vi "BasicFPGATest.vi"() -> ()   [LabVIEW 2015]
uses:
  Core/SingleAIConfig.ctl
  Core/ScaleAndLimitAI16Config.ctl
  Core/AI16LimitsConfig.ctl
  Core/AI16ScaleConfig.ctl
  <vilib>/Platform/TimedLoop/XDataNode/timing_clust.ctl
  <vilib>/Platform/TimedLoop/XDataNode/nitl_modes.ctl
  <vilib>/Platform/TimedLoop/XDataNode/wakeup.ctl
  <vilib>/rvi/Emulation/niFpgaGetClockAttributes.vi
  <vilib>/rvi/Emulation/niFpgaSctlEmulationGetInTimedLoop.vi
  <vilib>/rvi/Emulation/niFpgaEmulationReportErrorSimple.vi
  <vilib>/NI/PowerElectronicsControl/Utility/FPGA_Timers/TickTocks/Tick0.vi
  <vilib>/rvi/Emulation/niFpgaCriticalErrorInLSC.vi
  <vilib>/NI/PowerElectronicsControl/Utility/FPGA_Timers/TickTocks/Tock0.vi
  <vilib>/NI/PowerElectronicsControl/Utility/FPGA_Timers/TickTocks/Tick2.vi
  <vilib>/rvi/eio/common/nirviEmuTemplateMethod_errors.vi
  <vilib>/NI/PowerElectronicsControl/Utility/FPGA_Timers/TickTocks/Tock2.vi
  <vilib>/NI/PowerElectronicsControl/Utility/FPGA_Timers/TickTocks/Tick3.vi
  <vilib>/NI/PowerElectronicsControl/Utility/FPGA_Timers/TickTocks/Tock3.vi
  <vilib>/Platform/TimedLoop/XDataNode/XDataNode.xnode
  <vilib>/eio/EIONode/EIONode.xnode
  Core/ScaleAndLimit.lvlib
  <vilib>/Platform/TimedLoop/XDataNode/XDNodeRunTimeDep.lvlib
  <vilib>/NI/PowerElectronicsControl/Utility/FPGA_Timers/Timers.lvlib
panel:
  out "UnscaledAI":i16[](array[numeric])
  in  "DummyAI15":i16
  in  "SingleAIConfig":T1
  in  "loop wait":u32 caption="Count(Ticks)"
  out "scale and fault":u32
  out "I/O":u32
  in  "resetMaxTime":bool
  out "MaxTimes":u32[](array[numeric])
  out "Times":u32[](array[numeric])
  out "AILimitLow":u16 format="%.0x"
  out "AILimitHigh":u16 format="%.0x"
  out "AILimits":bool
  out "ScaledAI":sgl[](array[numeric])
  in  "ClearLimits":bool
  out "loop time":u32
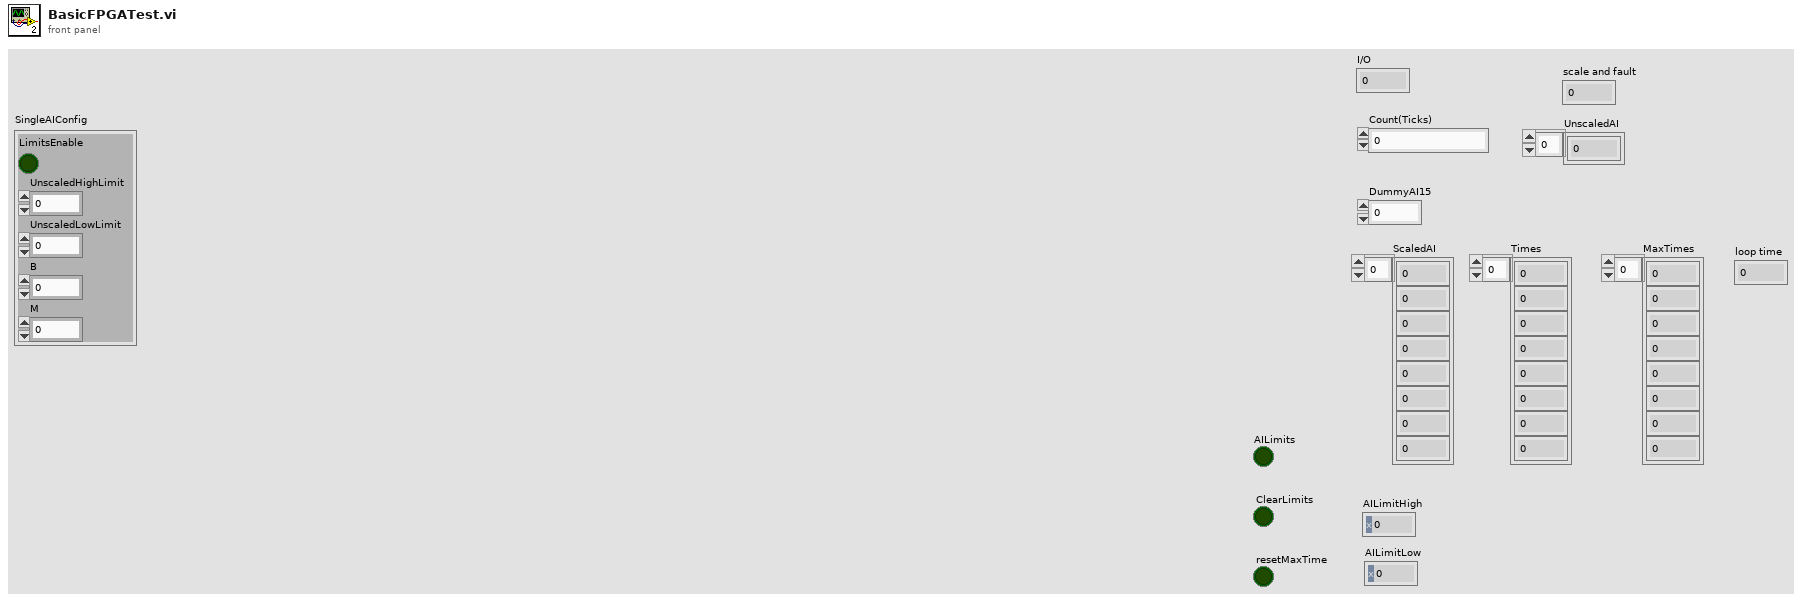
[diagram p1: front panel]
types:
  T1 = typedef "ScaleAndLimit.lvlib/SingleAIConfig.ctl" = cluster{"LimitsEnable":bool, "UnscaledHighLimit":i16, "UnscaledLowLimit":i16, "B":i16, "M":sgl}
  T2 = typedef "ScaleAndLimit.lvlib/ScaleAndLimitAI16Config.ctl" = cluster{"AI16Limits":T3, "AI16ScaleConfig":T4}
  T3 = typedef "ScaleAndLimit.lvlib/AI16LimitsConfig.ctl" = cluster{"LimitsEnabled":u16, "UnscaledHighLimit":i16[], "UnscaledLowLimit":i16[]}
  T4 = typedef "ScaleAndLimit.lvlib/AI16ScaleConfig.ctl" = cluster{"B":i16[], "M":sgl[]}
  T5 = typedef "Timers.lvlib/TimerRegisters.ctl" = cluster{"Tick0":refnum<k21>, "Tock0":refnum<k21>, "Tick1":refnum<k21>, "Tock1":refnum<k21>, "Tick2":refnum<k21>, "Tock2":refnum<k21>, "Tick3":refnum<k21>, "Tock3":refnum<k21>, "Tick4":refnum<k21>, "Tock4":refnum<k21>, "Tick5":refnum<k21>, "Tock5":refnum<k21>, "Tick6":refnum<k21>, "Tock6":refnum<k21>, "Tick7":refnum<k21>, "Tock7":refnum<k21>}
  T6 = typedef "XDNodeRunTimeDep.lvlib/timing_clust.ctl" = cluster{"Expected End [f-1]":u64, "Actual End [f-1]":u64, "Finished Late? [f-1]":bool, "Expected End [i-1]":u64, "Actual End [i-1]":u64, "Finished Late? [i-1]":bool, "Expected Start [i]":u64, "Actual Start [i]":u64, "Expected Start [f]":u64, "Actual Start [f]":u64, "Source Name":string, "Structure Name":string, "Period":i64, "Deadline":i64, "Offset":i64, "Start":i64, "Priority":i32, "Timeout":i32, "Mode":T7, "Wakeup Reason":T8, "Error":errorcluster, "Source Type":string, "Secondary Source Type":string, "Global End Time":u64, "Global Start Time":u64, "Frame Duration":u64, "Iteration Duration":u64, "Assigned CPU":i32, "I/O Scan Engine Mode":u32}
  T7 = typedef "XDNodeRunTimeDep.lvlib/nitl_modes.ctl" = enum32{"No Change", "Process missed periods, maintain original phase", "Discard missed periods, maintain original phase", "Process missed periods, ignore original phase", "Discard missed periods, ignore original phase"}
  T8 = typedef "XDNodeRunTimeDep.lvlib/wakeup.ctl" = enum32{"Normal", "Aborted", "Asynchronous wakeup", "Timing source error", "Timed loop error", "Timeout"}
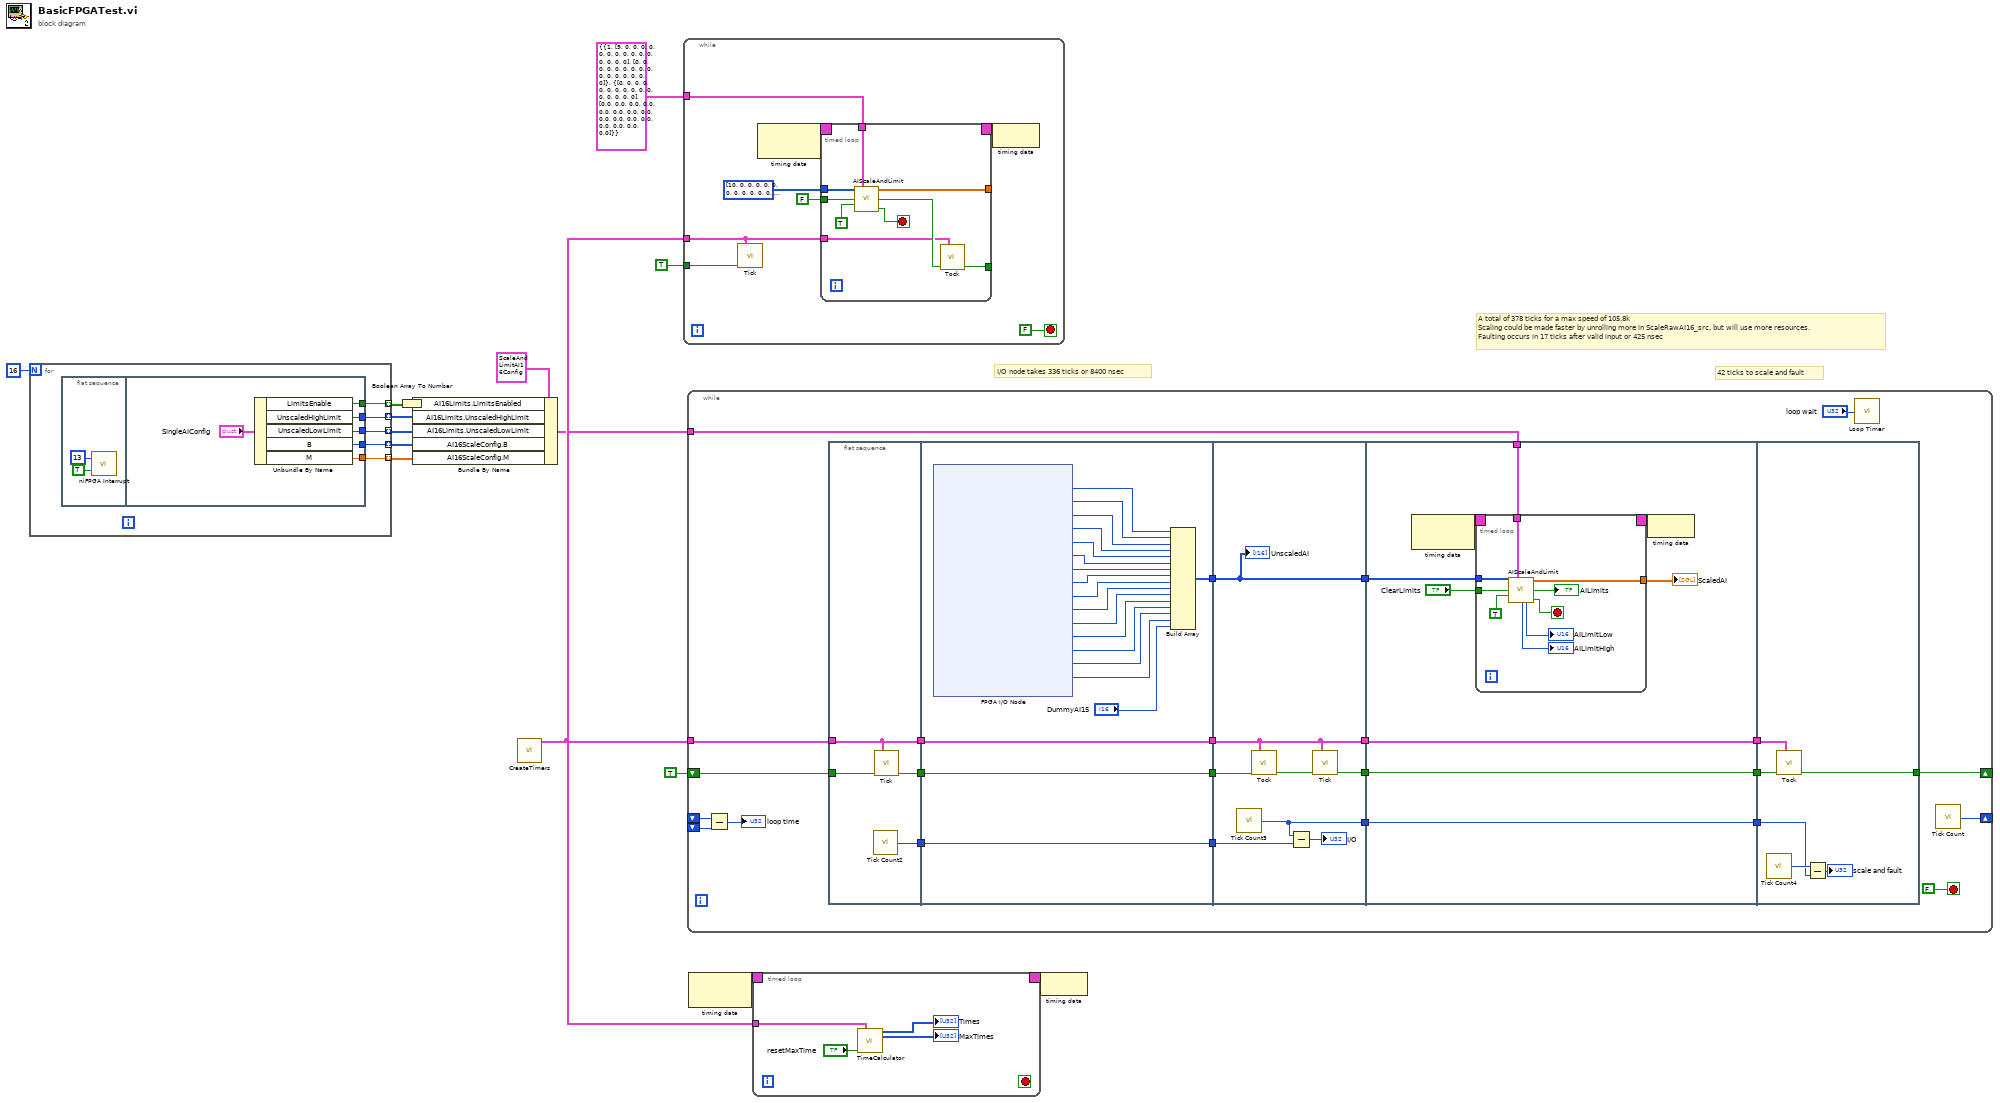
[diagram p0: block diagram]
diagram:
  # "A total of 378 ticks for a max speed of 105.8k\nScaling could be made faster by unrolling more in ScaleRawAI16_src, but will use more resources.\nFaulting occurs in 17 ticks after valid input or 425 nsec"
  # "42 ticks to scale and fault"
  # "I/O node takes 336 ticks or 8400 nsec"
  n1 = for {
    N: 16 -> [_]
    tunnel: [w20] -> w8 mode=indexing
    tunnel: [w19] -> w5 mode=indexing
    tunnel: [w18] -> w4 mode=indexing
    tunnel: [w17] -> w3 mode=indexing
    tunnel: [w16] -> w2 mode=indexing
    n2 = flat-sequence {
      tunnel: [w27] -> w20
      tunnel: [w26] -> w19
      tunnel: [w25] -> w18
      tunnel: [w24] -> w17
      tunnel: [w23] -> w16
      frame #0 {
        n3 = call <vilib>:"niFPGA Interrupt.vi"("Wait Until Cleared (F)"=TRUE, "IRQ Number (0)"=u8 13) -> ()  [unwired: 1 in]
      }
      frame #1 {
        n4 = Unbundle By Name("SingleAIConfig") -> ("LimitsEnable"=w27:bool, "UnscaledHighLimit"=w26:i16, "UnscaledLowLimit"=w25:i16, "B"=w24:i16, "M"=w23:sgl)
      }
    }
  }
  n5 = Boolean Array To Number(Boolean array=w8) -> (number=w6:u16)
  n6 = Bundle By Name(cluster=T2 {"AI16Limits"={"LimitsEnabled"=0, "UnscaledHighLimit"=[0, 0, 0, 0, 0, 0, 0, 0, 0, 0, 0, 0, 0, 0, 0, 0], "UnscaledLowLimit"=[0, 0, 0, 0, 0, 0, 0, 0, 0, 0, 0, 0, 0, 0, 0, 0]}, "AI16ScaleConfig"={"B"=[0, 0, 0, 0, 0, 0, 0, 0, 0, 0, 0, 0, 0, 0, 0, 0], "M"=[0.0, 0.0, 0.0, 0.0, 0.0, 0.0, 0.0, 0.0, 0.0, 0.0, 0.0, 0.0, 0.0, 0.0, 0.0, 0.0]}} ("AIConfig"), "AI16Limits.LimitsEnabled"=w6, "AI16Limits.UnscaledHighLimit"=w5, "AI16Limits.UnscaledLowLimit"=w4, "AI16ScaleConfig.B"=w3, "AI16ScaleConfig.M"=w2) -> (w1:T2)
  n7 = call <vilib>:"CreateTimers.vi"() -> ("TimerRegisters"=w10:T5)  [unwired: 15 in]
  n8 = while {
    tunnel: T2 {"AI16Limits"={"LimitsEnabled"=1, "UnscaledHighLimit"=[9, 0, 0, 0, 0, 0, 0, 0, 0, 0, 0, 0, 0, 0, 0, 0], "UnscaledLowLimit"=[0, 0, 0, 0, 0, 0, 0, 0, 0, 0, 0, 0, 0, 0, 0, 0]}, "AI16ScaleConfig"={"B"=[0, 0, 0, 0, 0, 0, 0, 0, 0, 0, 0, 0, 0, 0, 0, 0], "M"=[0.0, 0.0, 0.0, 0.0, 0.0, 0.0, 0.0, 0.0, 0.0, 0.0, 0.0, 0.0, 0.0, 0.0, 0.0, 0.0]}} ("RawAIConfig 2") -> [w33]
    tunnel: TRUE -> [w31]
    tunnel: w10 -> [w30]
    stop <- FALSE stop-if-true
    n9 = call-poly <vilib>:"Tick.vi"("TimerRegisters"=w30, "valid input"=w31) -> ()  [unwired: 13 in, 1 out]
    n10 = node-c288() -> (w36:T6)  [unwired: 1 in]
    n11 = timed-loop {
      timing: w36 -> [_]
      timing-out: [_] -> w35
      tunnel: i16[] [10, 0, 0, 0, 0, 0, 0, 0, 0, 0, 0, 0, 0, 0, 0, 0] -> [w45]
      tunnel: w33 -> [w44]
      tunnel: FALSE ("ClearFaults") -> [w43]
      tunnel: [w41] -> _
      tunnel: w30 -> [w38]
      tunnel: [w37] -> _
      stop <- w40 stop-if-true
      n12 = call "AIScaleAndLimit.vi"("UnscaledAI"=w45, "RawAIConfig"=w44, "ClearLimits"=w43, "input valid"=TRUE) -> ("ScaledAI"=w41:sgl[], "AILimits"=w39:bool, "output valid"=w40:bool)  [unwired: 6 in, 3 out]
      n13 = call-poly <vilib>:"Tock.vi"("TimerRegisters"=w38, "valid input"=w39) -> ("valid output"=w37:bool)  [unwired: 13 in]
    }
    n14 = node-c288(w35) -> ()
  }
  n15 = while {
    shift-right: [w72] -> _
    shift-left: _ -> [w71]
    shift-left: _ -> [w70]
    tunnel: w1 -> [w66]
    tunnel: w10 -> [w68]
    shift-right: [w52] -> _
    shift-left: TRUE ("valid input") -> [w55]
    stop <- FALSE stop-if-true
    n16 = Subtract(x=w71, y=w70) -> (x-y=→"loop time":u32)
    n17 = flat-sequence {
      tunnel: w68 -> [w77]
      tunnel: [w77] -> w61
      tunnel: [w76] -> w60
      tunnel: w55 -> [w75]
      tunnel: [w74] -> w54
      tunnel: [w82] -> w67
      tunnel: w61 -> [w82]
      tunnel: w60 -> [w81]
      tunnel: [w81] -> w59
      tunnel: w54 -> [w80]
      tunnel: [w80] -> w53
      tunnel: [w78] -> w51
      tunnel: w67 -> [w105]
      tunnel: [w105] -> w65
      tunnel: [w104] -> w62
      tunnel: w59 -> [w103]
      tunnel: [w101] -> w58
      tunnel: w53 -> [w100]
      tunnel: w51 -> [w98]
      tunnel: [w98] -> w50
      tunnel: w66 -> [w110]
      tunnel: w65 -> [w109]
      tunnel: [w109] -> w64
      tunnel: [w108] -> w63
      tunnel: w62 -> [w108]
      tunnel: w58 -> [w107]
      tunnel: [w107] -> w57
      tunnel: w50 -> [w106]
      tunnel: w64 -> [w133]
      tunnel: w63 -> [w132]
      tunnel: w57 -> [w130]
      tunnel: [w128] -> w52
      frame #0 {
        n18 = call "Tick Count2"() -> ("Tick Count(Ticks)"=w76:u32)
        n19 = call-poly <vilib>:"Tick.vi"("TimerRegisters"=w77, "valid input"=w75) -> ("valid output"=w74:bool)  [unwired: 13 in]
      }
      frame #1 {
        n20 = xnode "FPGA I/O Node"() -> ("RMC/Simultaneous/AI0"=w97:i16, "RMC/Simultaneous/AI1"=w96:i16, "RMC/Simultaneous/AI2"=w95:i16, "RMC/Simultaneous/AI3"=w94:i16, "RMC/Simultaneous/AI4"=w93:i16, "RMC/Simultaneous/AI5"=w92:i16, "RMC/Simultaneous/AI6"=w91:i16, "RMC/Simultaneous/AI7"=w90:i16, "RMC/Simultaneous/AI8"=w89:i16, "RMC/Simultaneous/AI9"=w88:i16, "RMC/Simultaneous/AI10"=w87:i16, "RMC/Simultaneous/AI11"=w86:i16, "RMC/Simultaneous/AI12"=w85:i16, "RMC/Simultaneous/AI13"=w84:i16, "RMC/Simultaneous/AI14"=w83:i16)  [unwired: 16 in, 17 out]
        n21 = Build Array(w97, w96, w95, w94, w93, w92, w91, w90, w89, w88, w87, w86, w85, w84, w83, "DummyAI15") -> (w78:i16[])
      }
      frame #2 {
        n22 = call "Tick Count3"() -> ("Tick Count(Ticks)"=w101:u32)
        n23 = call-poly <vilib>:"Tock.vi"("TimerRegisters"=w105, "valid input"=w100) -> ("valid output"=w99:bool)  [unwired: 13 in]
        n24 = Subtract(x=w101, y=w103) -> (x-y=→"I/O":u32)
        n25 = call-poly <vilib>:"Tick.vi"("TimerRegisters"=w105, "valid input"=w99) -> ("valid output"=w104:bool)  [unwired: 13 in]
        "UnscaledAI" <- w98
      }
      frame #3 {
        n26 = node-c288() -> (w114:T6)  [unwired: 1 in]
        n27 = timed-loop {
          timing: w114 -> [_]
          timing-out: [_] -> w113
          tunnel: w110 -> [w123]
          tunnel: "ClearLimits" -> [w122]
          tunnel: [w120] -> w112
          tunnel: w106 -> [w115]
          stop <- w118 stop-if-true
          n28 = call "AIScaleAndLimit.vi"("UnscaledAI"=w115, "RawAIConfig"=w123, "ClearLimits"=w122, "input valid"=TRUE) -> ("ScaledAI"=w120:sgl[], "AILimits"=→"AILimits":bool, "AILimitHigh"=→"AILimitHigh":u16, "ALimitLow"=→"AILimitLow":u16, "output valid"=w118:bool)  [unwired: 6 in, 1 out]
        }
        "ScaledAI" <- w112
        n29 = node-c288(w113) -> ()
      }
      frame #4 {
        n30 = call "Tick Count4"() -> ("Tick Count(Ticks)"=w131:u32)
        n31 = call-poly <vilib>:"Tock.vi"("TimerRegisters"=w133, "valid input"=w132) -> ("valid output"=w128:bool)  [unwired: 13 in]
        n32 = Subtract(x=w131, y=w130) -> (x-y=→"scale and fault":u32)
      }
    }
    n33 = call "Loop Timer"("Count(Ticks)"="loop wait") -> ()  [unwired: 1 out]
    n34 = call "Tick Count"() -> ("Tick Count(Ticks)"=w72:u32)
  }
  n35 = node-c288() -> (w15:T6)  [unwired: 1 in]
  n36 = timed-loop {
    timing: w15 -> [_]
    timing-out: [_] -> w14
    tunnel: w10 -> [w137]
    stop <- _ stop-if-true
    n37 = call <vilib>:"TimeCalculator.vi"("TimerRegisters"=w137, "resetMaxTime"="resetMaxTime") -> ("Times"=→"Times":u32[], "MaxTimes"=→"MaxTimes":u32[])  [unwired: 12 in]
  }
  n38 = node-c288(w14) -> ()
